vi "fftw__destroy_plan_poly.vi"   [LabVIEW 2020, in "FFTWDLL.lvlib"]
doc: "Destroy FFTW plan."
uses:
  FFTWDLL.lvlib
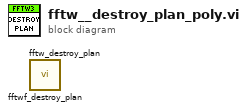
[diagram p0: block diagram]
diagram:
  n1 = call "fftwf_destroy_plan.vi"() -> ()  [unwired: 11 in, 1 out]
  n2 = call "fftw_destroy_plan.vi"() -> ()  [unwired: 11 in, 1 out]
